vi "Simulation Full Step.vi"(8 "Error In":errorcluster, 10 "Play Button (false)":bool, 11 "simulator":T3={"configuration"={"maxTime"=5.0, "enableVisualization"=TRUE, "Environment Definition"=path "iRobot Navigation State Machine.vi", "Record Location"=path "Simulation Record.xml", "autograde?"=TRUE, "interactive?"=FALSE, "Feedback Mode"=enum."debug navigation", "Robot State Charts"=[path "C:/Users/blueuser/Desktop/Robo Sim Berkley/cpsgrader-release-0.4/Simulators/EECS149lab/src/LabVIEW/statechart/Simulation Statechart.vi"], "statechart"=path "C:/Users/blueuser/Desktop/Robo Sim Berkley/cpsgrader-release-0.4/Simulators/EECS149lab/src/LabVIEW/statechart/Simulation Statechart.vi"}, "Statechart\ndisplay"=refnum, "first step?"=FALSE, "Robots Simulation Statecharts"=[], "Robots"=[]}) -> (0 "Error Out":errorcluster, 1 "continue to next step?":bool, 2 "simulated time (s)":sgl format="%7.3g", 3 "simulator":T3={"configuration"={"maxTime"=5.0, "enableVisualization"=TRUE, "Environment Definition"=path "iRobot Navigation State Machine.vi", "Record Location"=path "Simulation Record.xml", "autograde?"=TRUE, "interactive?"=FALSE, "Feedback Mode"=enum."debug navigation", "Robot State Charts"=[path "C:/Users/blueuser/Desktop/Robo Sim Berkley/cpsgrader-release-0.4/Simulators/EECS149lab/src/LabVIEW/statechart/Simulation Statechart.vi"], "statechart"=path "C:/Users/blueuser/Desktop/Robo Sim Berkley/cpsgrader-release-0.4/Simulators/EECS149lab/src/LabVIEW/statechart/Simulation Statechart.vi"}, "Statechart\ndisplay"=refnum, "first step?"=FALSE, "Robots Simulation Statecharts"=[], "Robots"=[]}, 5 "Kobuki Sensors Display":T1 {"Right Wheel (mm/s)" scale=-500.0..500.0; "Left Wheel (mm/s)" scale=-500.0..500.0})   [LabVIEW 2015]
uses:
  Simulator.ctl
  CyberSim interface/Simulation Configuration.ctl
  autograder/feedbackMode.ctl
  Multi Bot Code/RobotData.ctl
  <instrlib>/DC Motor Controller/HAIOL/DC Motor Controller.lvclass
  shared/Kobuki Sensor Display.ctl
  Simulation Call Statechart Operation.ctl
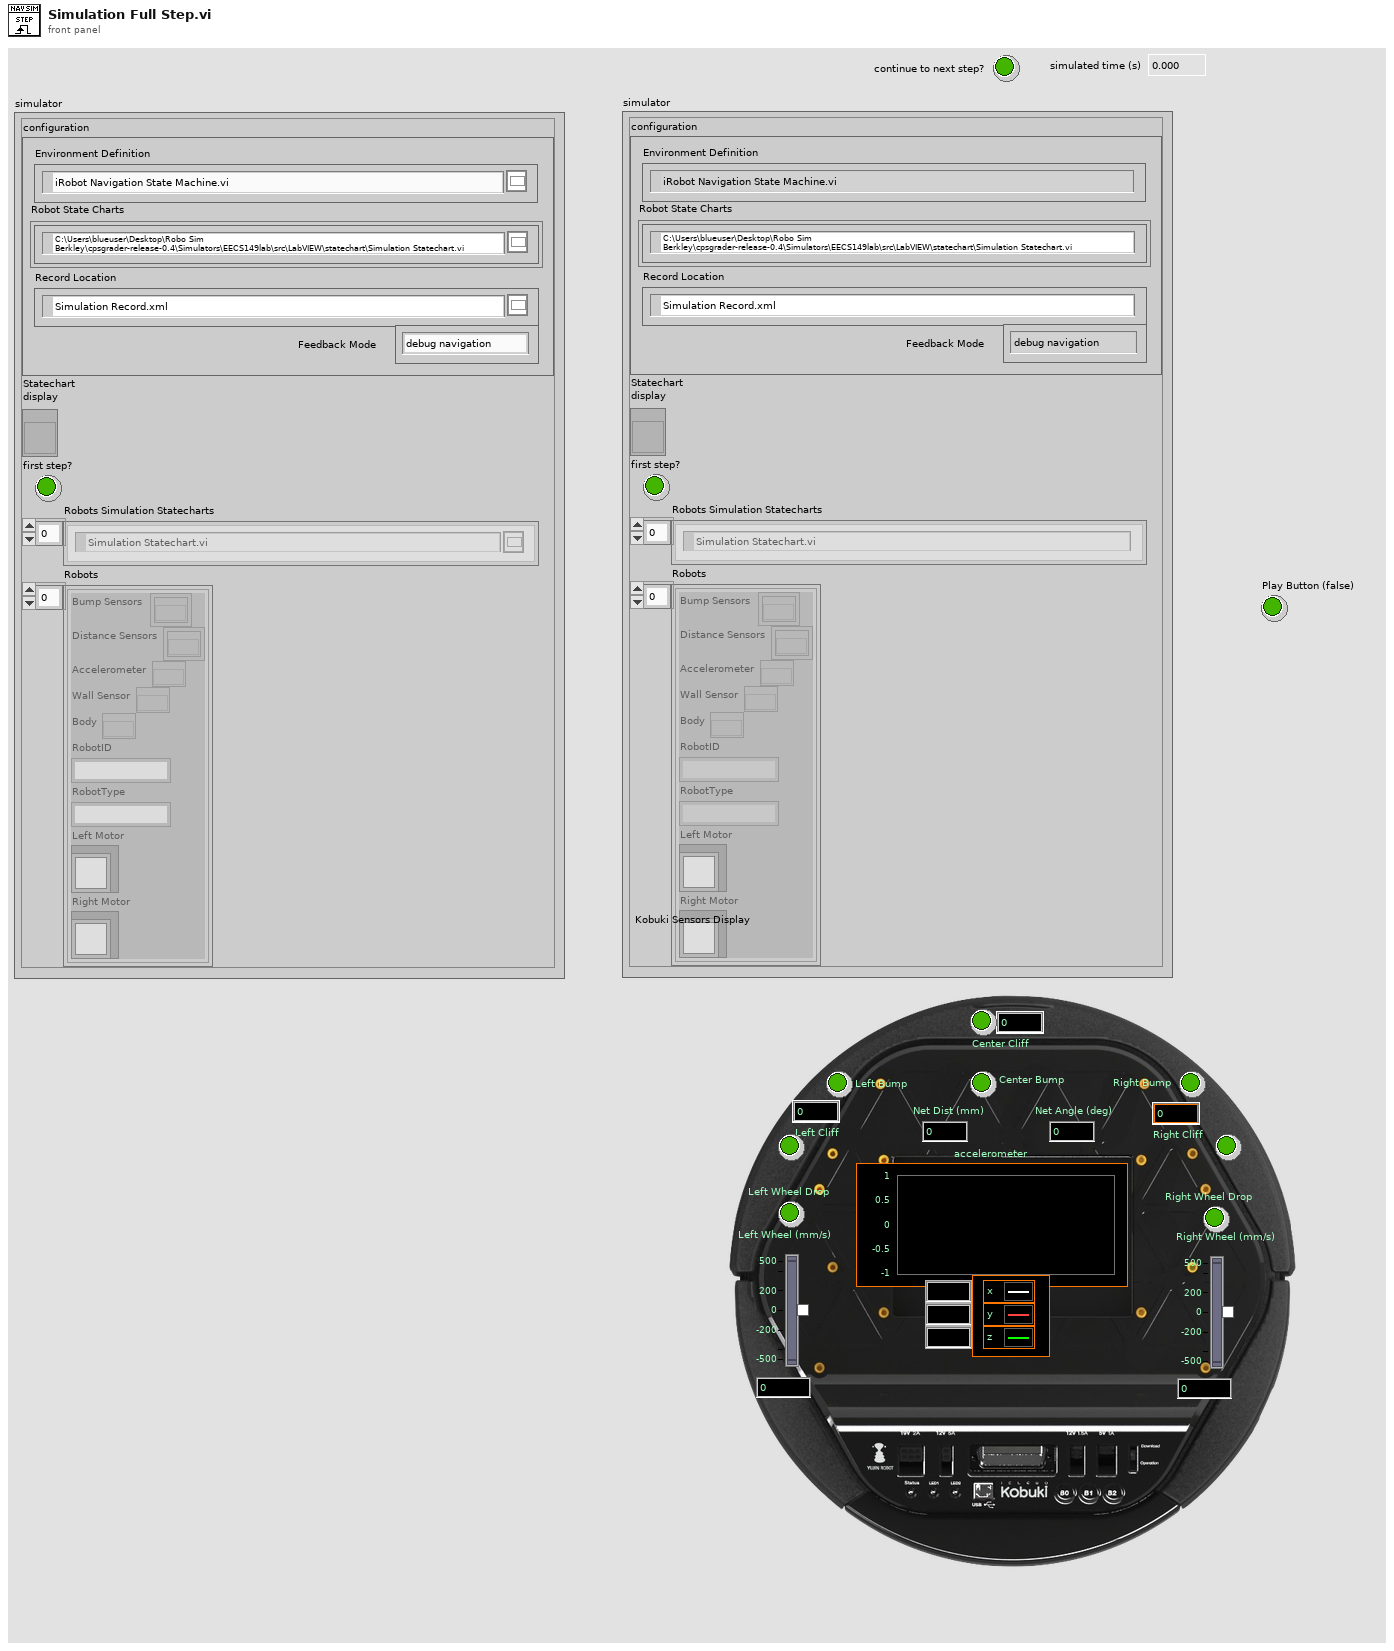
[diagram p1: front panel]
types:
  T1 = typedef "Kobuki Sensor Display.ctl" = cluster{"Center Bump":bool, "Left Wheel Drop":bool, "Right Wheel Drop":bool, "Left Bump":bool, "Right Bump":bool, "Left Cliff":bool, "Center Cliff":bool, "Right Cliff":bool, "Net Dist (mm)":i32, "Net Angle (deg)":i32, "Left Cliff":u16, "Center Cliff":u16, "Right Cliff":u16, "  Left Wheel (mm/s)":i16, "Right Wheel (mm/s)":i16, "accelerometer":T2}
  T2 = typedef "Accelerometer.ctl" = cluster{"x axis (g)":dbl, "y axis (g)":dbl, "z axis (g)":dbl}
  T3 = typedef "Simulator.ctl" = cluster{"configuration":T4, "Statechart\ndisplay":refnum<vi>, "first step?":bool, "Robots Simulation Statecharts":path[], "Robots":T6[]}
  T4 = typedef "Simulation Configuration.ctl" = cluster{"maxTime":sgl, "enableVisualization":bool, "Environment Definition":path, "Record Location":path, "autograde?":bool, "interactive?":bool, "Feedback Mode":T5, "Robot State Charts":path[], "statechart":path}
  T5 = typedef "feedbackMode.ctl" = enum32{"debug navigation", "debug hill climb", "autograde navigation", "autograde hill climb"}
  T6 = typedef "RobotData.ctl" = cluster{"Bump Sensors":refnum<k20>[], "Distance Sensors":refnum<k20>[], "Accelerometer":refnum<k20>, "Wall Sensor":refnum<k20>, "Body":refnum<k20>, "RobotID":string, "RobotType":string, "Left Motor":refnum<class "DC Motor Controller.lvclass">, "Right Motor":refnum<class "DC Motor Controller.lvclass">}
  T7 = typedef "Simulation Call Statechart Operation.ctl" = enum16{"Initialize", "Call Statechart", "Finalize"}
  T8 = typedef "Sensors.ctl" = cluster{"net distance (mm)":i32, "net angle (deg)":i32, "accelerometer":T2, "Is Simulator?":bool, "Kobuki Sensors":T9, "Requested Left Wheel Velocity(mm/s)":i32, "Requested Right Wheel Velocity(mm/s)":i32}
  T9 = typedef "KobukiSensors.ctl" = cluster{"Bumps + Wheel Drops":T10, "Cliff Left":bool, "Cliff Center":bool, "Cliff Right":bool, "Cliff Left Signal":u16, "Cliff Center Signal":u16, "Cliff Right Signal":u16, "Buttons":T11, "Left Wheel Encoder (ticks)":u16, "Right Wheel Encoder (ticks) ":u16, "Left  Wheel PWM":i8, "Right Wheel PWM":i8, "Left Wheel OverCurrent":bool, "Right Wheel OverCurrent ":bool, "Right Wheel Current (x10mA)":i16, "Left  Wheel Current  (x10mA)":i16, "TimeStamp":u16, "Battery Voltage (mV)":i16, "Angle( of 100deg)":i16, "Angle Rate( of 100 deg/sec)":i16, "Charger Source ":i8}
  T10 = typedef "Kobuki Bumps and WheelDrops.ctl" = cluster{"Wheeldrop Left":bool, "Wheeldrop Right":bool, "Bump Left":bool, "Bump Center":bool, "Bump Right":bool}
  T11 = typedef "Kobuki Buttons.ctl" = cluster{"B0":bool, "B1":bool, "B2":bool}
  T12 = typedef "Simulation Trace Element.ctl" = cluster{"sensors":T8, "position":T13, "orientation":T14, "Simulation Time (s)":sgl}
  T13 = typedef "Simulated Position.ctl" = cluster{"x (m)":sgl, "y (m)":sgl, "z (m)":sgl}
  T14 = typedef "Simulated Orientation.ctl" = cluster{"roll (deg)":sgl, "pitch (deg)":sgl, "yaw (deg)":sgl}
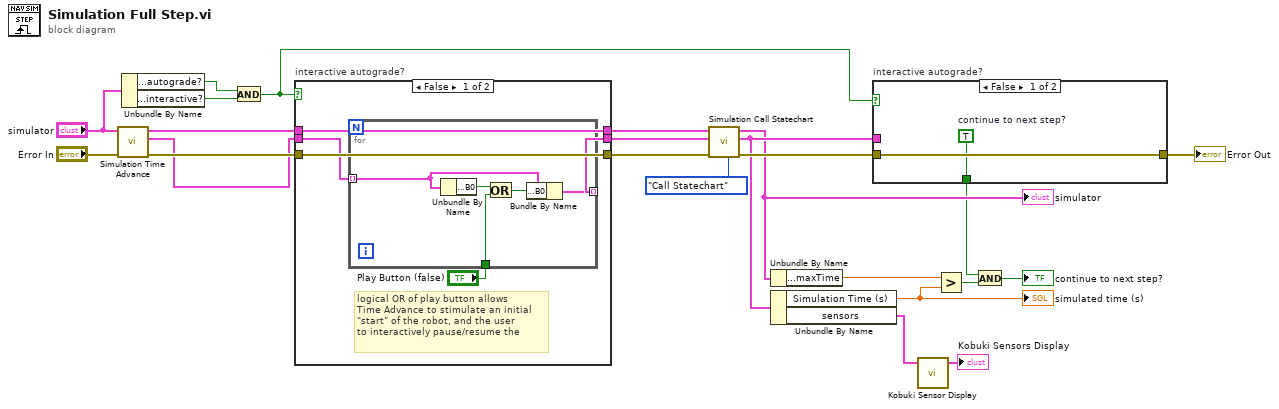
[diagram p0: block diagram]
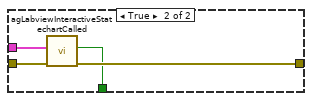
[diagram p2: hidden frame]
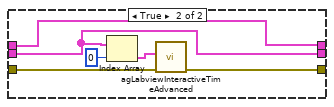
[diagram p3: hidden frame]
diagram:
  n1 = call "Simulation Time Advance.vi"("error in (no error)"="Error In", "simulator"="simulator") -> ("error out"=w15:errorcluster, "Robot Sensors"=w3:T8[], "simulator"=w16:T3)  [unwired: 7 in]
  n2 = Unbundle By Name("simulator") -> ("configuration.autograde?"=w18:bool, "configuration.interactive?"=w17:bool)
  n3 = And(x=w18, y=w17) -> (x .and. y?=w11:bool)
  n4 = case "interactive autograde?" shown="False" w11 {
    tunnel: w16 -> [w27 w38]
    tunnel: w3 -> [w25 w34]
    tunnel: w15 -> [w26 w39]
    tunnel: [w27 w38] -> w14
    tunnel: [w24 w34] -> w13
    tunnel: [w26 w37] -> w12
    frame False {
      # "logical OR of play button allows\nTime Advance to stimulate an initial\n\"start\" of the robot, and the user\nto interactively pause/resume the"
      n5 = for {
        tunnel: "Play Button (false)" -> [w29]
        tunnel: w25 -> [w30] mode=indexing
        tunnel: [w33] -> w24 mode=indexing
        n6 = Unbundle By Name(w30) -> ("Kobuki Sensors.Buttons.B0"=w31:bool)
        n7 = Or(x=w31, y=w29) -> (x .or. y?=w32:bool)
        n8 = Bundle By Name(cluster=w30, "Kobuki Sensors.Buttons.B0"=w32) -> (w33:T8)
      }
    }
    frame True {
      n9 = Index Array(array=w34, index=0) -> (element=w35:T8)
      n10 = call "agLabviewInteractiveTimeAdvanced.vi"("Error In"=w39, "sensors"=w35) -> ("Error Out"=w37:errorcluster)  [unwired: 8 in, 1 out]
    }
  }
  n11 = call "Simulation Call Statechart.vi"("operation"=Simulation_Call_Statechart_Operation."Call Statechart", "error in"=w12, "Multi Bot Sensors"=w13, "simulator"=w14) -> ("error out"=w10:errorcluster, "trace element"=w9:T12, "simulator"=w7:T3)  [unwired: 5 in]
  "simulator" <- w7
  n12 = Unbundle By Name(w7) -> ("configuration.maxTime"=w22:sgl)
  n13 = Unbundle By Name(w9) -> ("Simulation Time (s)"=w21:sgl, "sensors"=w1:T8)
  "simulated time (s)" <- w21
  n14 = case "interactive autograde?" shown="False" w11 {
    tunnel: w10 -> [w41 w45]
    tunnel: w9 -> [_ w44]
    tunnel: [w41 w43] -> w8
    tunnel: [w40 w42] -> w5
    frame False {
      w40 = TRUE  # continue to next step?
    }
    frame True {
      n15 = call "agLabviewInteractiveStatechartCalled.vi"("Error In"=w45, "Trace Element"=w44) -> ("Error Out"=w43:errorcluster, "continue to next step?"=w42:bool)  [unwired: 8 in]
    }
  }
  "Error Out" <- w8
  n16 = call "Kobuki Sensor Display.vi"("sensors"=w1) -> ("Kobuki Sensors Display"=→"Kobuki Sensors Display":T1)  [unwired: 4 in]
  n17 = Greater?(x=w22, y=w21) -> (0:w6:bool)
  n18 = And(x=w5, y=w6) -> (x .and. y?=→"continue to next step?":bool)
